vi "comaparator.vi"() -> ()   [LabVIEW 2019]
panel:
  in  "error in (no error)":errorcluster
  out "error out":errorcluster
  out "String":string
  out "Current row":i32
  out "Array":string[](array[string])
  in  "File A":path
  in  "File B":path
  in  "milliseconds to wait":u32=2000
  out "Row of Value-sets out of range":i32[](array[numeric])
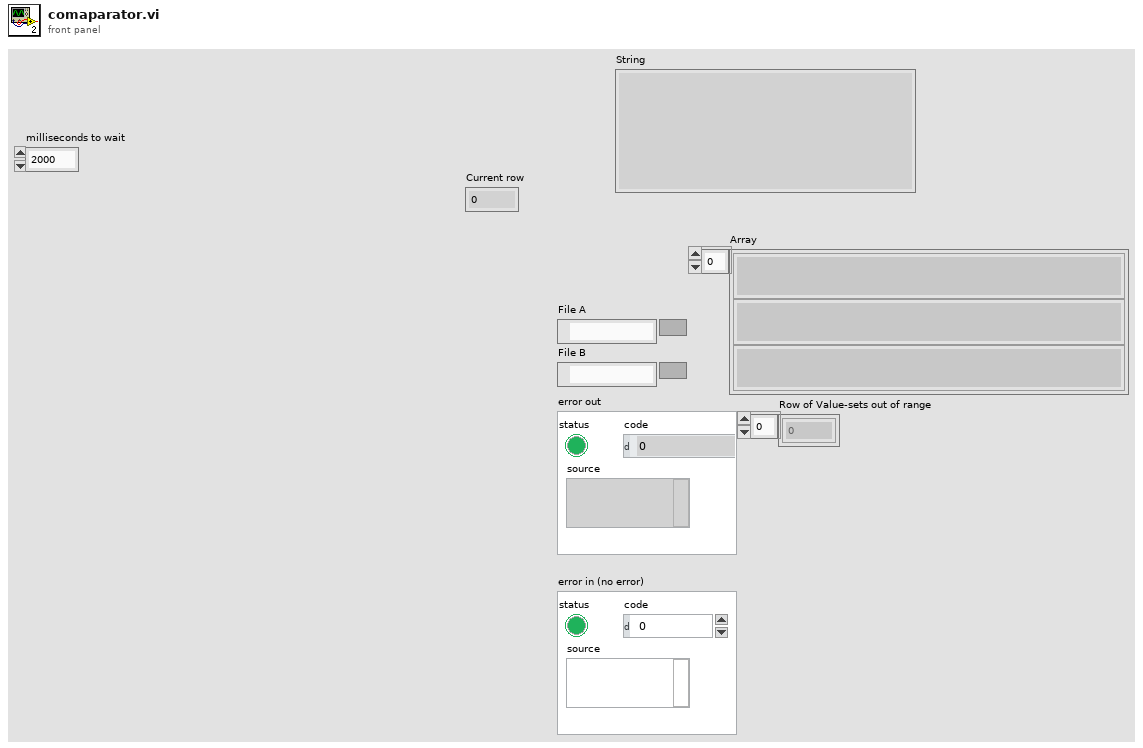
[diagram p1: front panel]
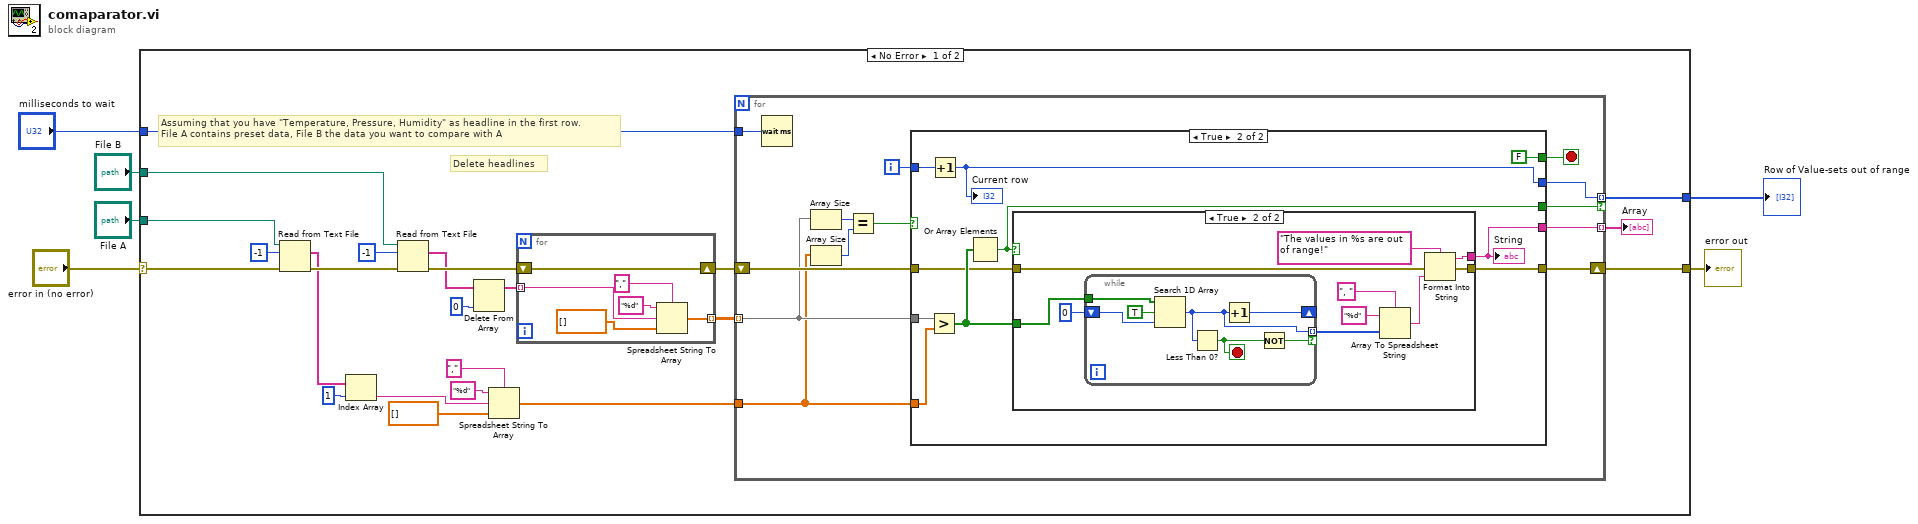
[diagram p0: block diagram]
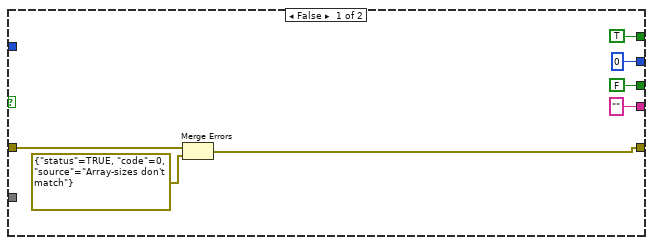
[diagram p2: hidden frame]
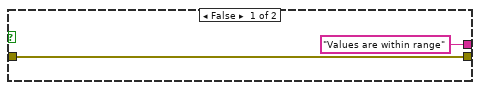
[diagram p3: hidden frame]
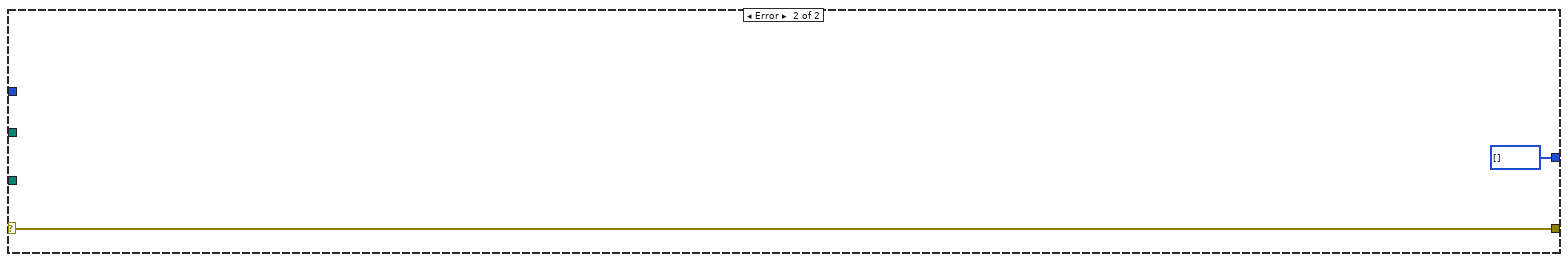
[diagram p4: hidden frame]
diagram:
  n1 = case shown="No Error" "error in (no error)" {
    selector: "error in (no error)" -> [w25 w86]
    tunnel: [w12 w86] -> w5
    tunnel: "File A" -> [w29 _]
    tunnel: "File B" -> [w28 _]
    tunnel: "milliseconds to wait" -> [w13 _]
    tunnel: [w7 i32[] []] -> w1
    frame No Error {
      # "Delete headlines"
      # "Assuming that you have \"Temperature, Pressure, Humidity\" as headline in the first row.\nFile A contains preset data, File B the data you want to compare with A"
      n2 = Read from Text File(file (use dialog)=w29, count=-1, error in=w25) -> (text=w22:string[], error out=w24:errorcluster)  [unwired: 1 in, 2 out]
      n3 = Index Array(array=w22, index=1) -> (element=w19:string)
      n4 = Read from Text File(file (use dialog)=w28, count=-1, error in=w24) -> (text=w11:string[], error out=w15:errorcluster)  [unwired: 1 in, 2 out]
      n5 = Delete From Array(array=w11, index=0) -> (array with subset deleted=w9:string[])  [unwired: 1 in, 1 out]
      n6 = Spreadsheet String To Array(delimiter (Tab)=",", format string="%d", spreadsheet string=w19, array type (2D Dbl)=dbl[] []) -> (array=w16:dbl[])
      n7 = for {
        tunnel: w9 -> [w81] mode=indexing
        tunnel: [w80] -> w17 mode=indexing
        shift-right: [w79] -> w14
        shift-left: w15 -> [w79]
        n8 = Spreadsheet String To Array(delimiter (Tab)=",", format string="%d", spreadsheet string=w81, array type (2D Dbl)=dbl[] []) -> (array=w80:dbl[])
      }
      n9 = for {
        tunnel: w17 -> [w35] mode=indexing
        tunnel: w16 -> [w34]
        shift-right: [w40] -> w12
        shift-left: w14 -> [w42]
        tunnel: w13 -> [w41]
        tunnel: [w38] -> w8 mode=indexing
        tunnel: [w37] -> w7 mode=indexing if=w36
        i -> [w39]
        stop <- w30 stop-if-true
        n10 = Wait (ms)(milliseconds to wait=w41) -> ()  [unwired: 1 out]
        n11 = Array Size(array=w35) -> (size(s)=w33:i32)
        n12 = Array Size(array=w34) -> (size(s)=w32:i32)
        n13 = Equal?(x=w33, y=w32) -> (x = y?=w31:bool)
        n14 = case shown="True" w31 {
          tunnel: w42 -> [w48 w58]
          tunnel: [w47 w57] -> w40
          tunnel: w39 -> [_ w56]
          tunnel: ["" w55] -> w38
          tunnel: [0 w54] -> w37
          tunnel: [FALSE w53] -> w36
          tunnel: w35 -> [_ w52]
          tunnel: w34 -> [_ w51]
          tunnel: [TRUE FALSE] -> w30
          frame False {
            n15 = Merge Errors(w48, errorcluster {"status"=TRUE, "code"=0, "source"="Array-sizes don't match"} ("error constant")) -> (w47:errorcluster)
          }
          frame True {
            n16 = Greater?(x=w52, y=w51) -> (0:w59:bool[])
            n17 = Increment(x=w56) -> (x+1=w54:i32)
            "Current row" <- w54
            n18 = Or Array Elements(Boolean array=w59) -> (logical OR=w53:bool)
            n19 = case shown="True" w53 {
              tunnel: w59 -> [_ w71]
              tunnel: w58 -> [w61 w65]
              tunnel: [w61 w64] -> w57
              tunnel: ["Values are within range" w62] -> w55
              frame False {
              }
              frame True {
                n20 = while {
                  tunnel: w71 -> [w78]
                  shift-right: [w74] -> _
                  shift-left: 0 -> [w76]
                  tunnel: [w75] -> w69 mode=indexing if=w72
                  stop <- w73 stop-if-true
                  n21 = Search 1D Array(1D array=w78, element=TRUE, start index (0)=w76) -> (index of element=w75:i32)
                  n22 = Less Than 0?(x=w75) -> (x < 0?=w73:bool)
                  n23 = Increment(x=w75) -> (x+1=w74:i32)
                  n24 = Not(x=w73) -> (.not. x?=w72:bool)
                }
                n25 = Array To Spreadsheet String(delimiter (Tab)=", ", array=w69, 3:"%d" ("format string")) -> (spreadsheet string=w66:string)
                n26 = Format Into String(format string="The values in %s are out of range!" ("initial string"), error in=w65, w66) -> (resulting string=w62:string, error out=w64:errorcluster)  [unwired: 1 in]
              }
            }
            "String" <- w55
          }
        }
      }
      "Array" <- w8
    }
    frame Error {
    }
  }
  "error out" <- w5
  "Row of Value-sets out of range" <- w1
